vi "Log State.vi"(8 "error in (no error)":errorcluster, 11 "Framework in":refnum<class "Framework.lvclass">) -> (0 "error out":errorcluster, 3 "Framework out":refnum<class "Framework.lvclass">)   [LabVIEW 2019, in "DSF Core.lvlib" / "Framework.lvclass"]
uses:
  Framework.lvclass
  Framework.lvclass/Framework.ctl
  <vilib>/NI/Memory Manager/Classes/Pointer/Pointer.lvclass/Pointer.ctl
  Interface/Logging/Command Data.ctl
  Interface/Logging/Command.ctl
  Interface/Logging/Parameters.ctl
  Interface/Logging/Framework State Parameters.ctl
  Framework States.ctl
  Pointers/Error/Error Pointer.lvclass
  C:/Program Files (x86)/National Instruments/LabVIEW 2019/vi.lib/NI/Memory Manager/Classes/Pointer/Pointer.lvclass
  Interface/Logging/Send Logging Command.vi
  Interface/Logging/Logging Interface.lvclass
  <vilib>/NI/Memory Manager/Classes/Pointer/Pointer.lvclass
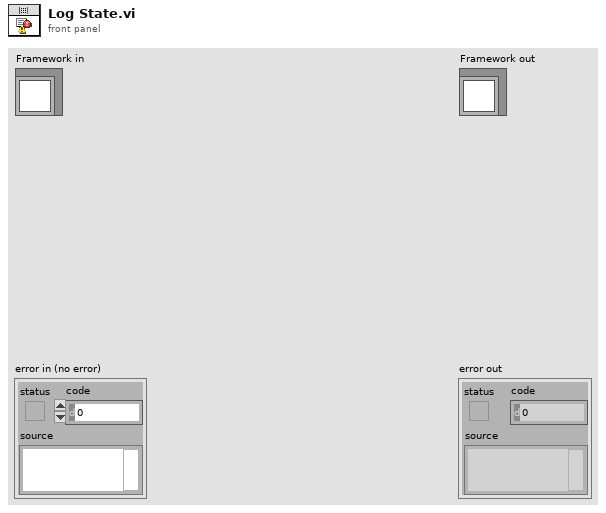
[diagram p1: front panel]
types:
  T1 = typedef "DSF Core.lvlib/Framework.lvclass/Framework States.ctl" = enum8{"Uninitialized", "Initialized", "Start", "Rx", "Tx", "Shutdown"}
  T2 = typedef "DSF Core.lvlib/Logging Interface.lvclass/Parameters.ctl" = cluster{"arg1":u64, "arg2":u64}
  T3 = typedef "DSF Core.lvlib/Logging Interface.lvclass/Framework State Parameters.ctl" = cluster{"state":T1, "unused":u8, "unused 2":u16, "unused 3":u32, "error pointer":u64}
  T4 = typedef "DSF Core.lvlib/Logging Interface.lvclass/Command.ctl" = enum8{"Idle", "Start", "Log Framework State", "Log Plugin State", "Log Dispatcher State", "Shutdown"}
  T5 = typedef "DSF Core.lvlib/Logging Interface.lvclass/Command Data.ctl" = cluster{"Command":T4, "Parameters":T2}
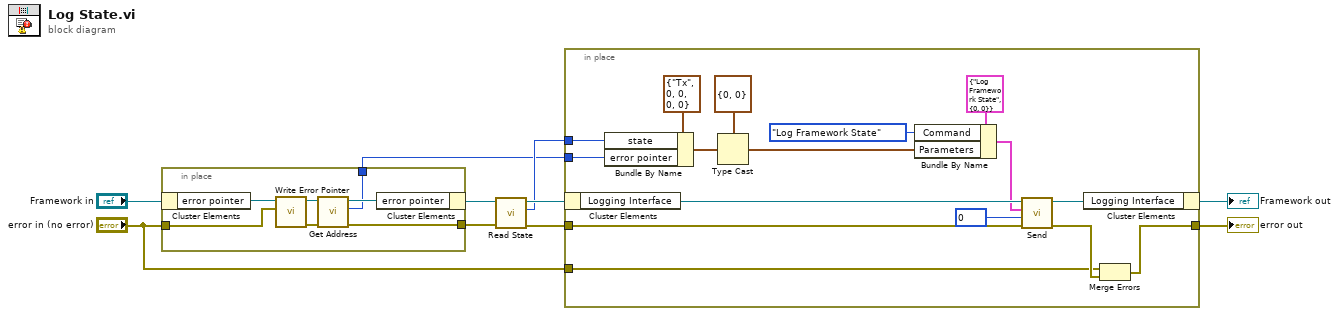
[diagram p0: block diagram]
diagram:
  n1 = in-place {
    in-place-border: "error in (no error)" -> [w11]
    in-place-border: [w15] -> w4
    in-place-border: [w12] -> w2
    n2 = in-place-cluster #1("Framework in") -> ("error pointer"=w16:refnum<class "Error Pointer.lvclass">)
    n3 = call "Write Error Pointer.vi"("error"=w11, "Error Pointer in"=w16) -> ("error out"=w15:errorcluster, "Error Pointer in"=w14:refnum<class "Error Pointer.lvclass">)  [unwired: 8 in]
    n4 = call <vilib>:"Get Address.vi"("Pointer in"=w14) -> ("address"=w12:u64, "Pointer out"=w13:refnum<class "Error Pointer.lvclass">)  [unwired: 9 in]
    n5 = in-place-cluster #1("error pointer"=w13) -> (w3:refnum<class "Framework.lvclass">)
  }
  n6 = call "Read State.vi"("error in (no error)"=w4, "Framework in"=w3) -> ("error out"=w8:errorcluster, "state"=w6:T1, "Framework out"=w7:refnum<class "Framework.lvclass">)  [unwired: 7 in]
  n7 = in-place {
    in-place-border: [w20] -> w10
    in-place-border: w8 -> [w18]
    in-place-border: w6 -> [w22]
    in-place-border: w2 -> [w21]
    in-place-border: "error in (no error)" -> [w17]
    n8 = in-place-cluster #2(w7) -> ("Logging Interface"=w32:refnum<class "Logging Interface.lvclass">)
    n9 = Bundle By Name(cluster=T3 {"state"=enum."Tx", "unused"=0, "unused 2"=0, "unused 3"=0, "error pointer"=0} ("Parameters"), "state"=w22, "error pointer"=w21) -> (w27:T3)
    n10 = Type Cast(type=T2 {"arg1"=0, "arg2"=0} ("Parameters"), x=w27) -> (*(type *) &x=w25:T2)
    n11 = Bundle By Name(cluster=T5 {"Command"=enum."Log Framework State", "Parameters"={"arg1"=0, "arg2"=0}} ("command"), "Command"=Command."Log Framework State", "Parameters"=w25) -> (w23:T5)
    n12 = call-poly "Send.vi"("error in (no error)"=w18, "timeout in ms (0)"=0, "command"=w23, "Logging Interface in"=w32) -> ("error out"=w19:errorcluster, "Logging Interface out"=w29:refnum<class "Logging Interface.lvclass">)  [unwired: 6 in]
    n13 = in-place-cluster #2("Logging Interface"=w29) -> (→"Framework out":refnum<class "Framework.lvclass">)
    n14 = Merge Errors(w17, w19) -> (w20:errorcluster)
  }
  "error out" <- w10
